vi "create list of values to scan.vi"() -> ()   [LabVIEW 2020]
uses:
  scan parameters.ctl
  d18e9d24-9158-4411-aad9-bee36d7b6cc6.vi
panel:
  out "shot values":dbl[](graph)
  in  "Scan parameters":T1 {"Scan Start" format="%#.9p"; "Scan End" format="%#.9p"; "Scan Step Size" format="%#.9p"}
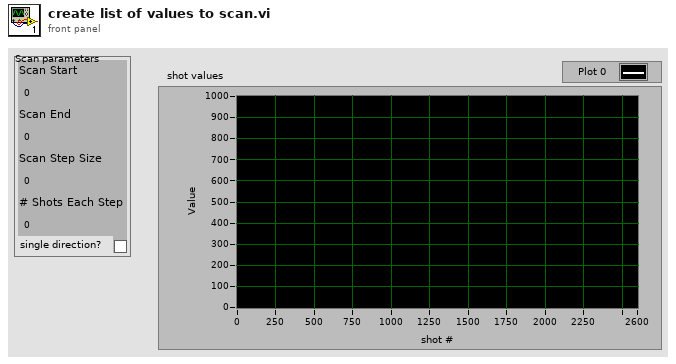
[diagram p1: front panel]
types:
  T1 = typedef "scan parameters.ctl" = cluster{"Scan Start":dbl, "Scan End":dbl, "Scan Step Size":dbl, "# Shots Each Step":u32, "single direction?":bool}
  T2 = enum32{"Single parameter scan", "Multi parameter scan"}
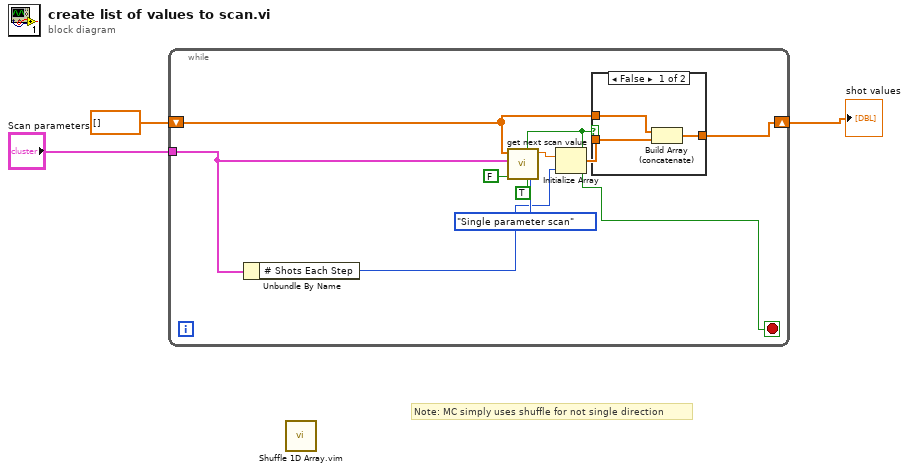
[diagram p0: block diagram]
diagram:
  # "Note: MC simply uses shuffle for not single direction"
  n1 = while {
    tunnel: "Scan parameters" -> [w6]
    shift-right: [w9] -> w1
    shift-left: dbl[] [] ("parameter vals scanned") -> [w10]
    stop <- w8 stop-if-true
    n2 = Unbundle By Name(w6) -> ("# Shots Each Step"=w5:u32)
    n3 = call "get next scan value.vi"("File scan type"=T2."Single parameter scan", "Scan(T) or NoScan"=TRUE, "File Scan"=FALSE, "Scan parameters"=w6, "parameter vals scanned"=w10) -> ("next value"=w7:dbl, "quit"=w8:bool)  [unwired: 4 in, 1 out]
    n4 = Initialize Array(w7, w5) -> (w4:dbl[])
    n5 = case shown="False" w8 {
      tunnel: w10 -> [w16 w17]
      tunnel: w4 -> [w15 _]
      tunnel: [w14 w17] -> w9
      frame False {
        n6 = Build Array (concatenate)(w16, w15) -> (w14:dbl[])
      }
      frame True {
      }
    }
  }
  "shot values" <- w1
  n7 = call "Shuffle 1D Array.vim"() -> ()  [unwired: 5 in, 1 out]
